vi "Day 8 - Haunted Wasteland.vi"() -> ()   [LabVIEW 2020, in "AoC 2023.lvlib"]
uses:
  AoC 2023.lvlib
  0a6171a5-c240-4508-9ae7-3547d43446d7.vi
  <vilib>/gmath/NI_AAL_MathFunc.lvlib
panel:
  out "Puzzle Part-2 Answer":string
  out "Puzzle Answer":string
  in  "Puzzle Input":string="RL\n\nAAA = (BBB, CCC)\nBBB = (DDD, EEE)\nCCC = (ZZZ, GGG)\nDDD = (DDD, DDD)\nEEE = (EEE, EEE)\nGGG = (GGG, GGG)\nZZZ = (ZZZ, ZZZ)"
  # "Enter the Puzzle Input and run the VI"
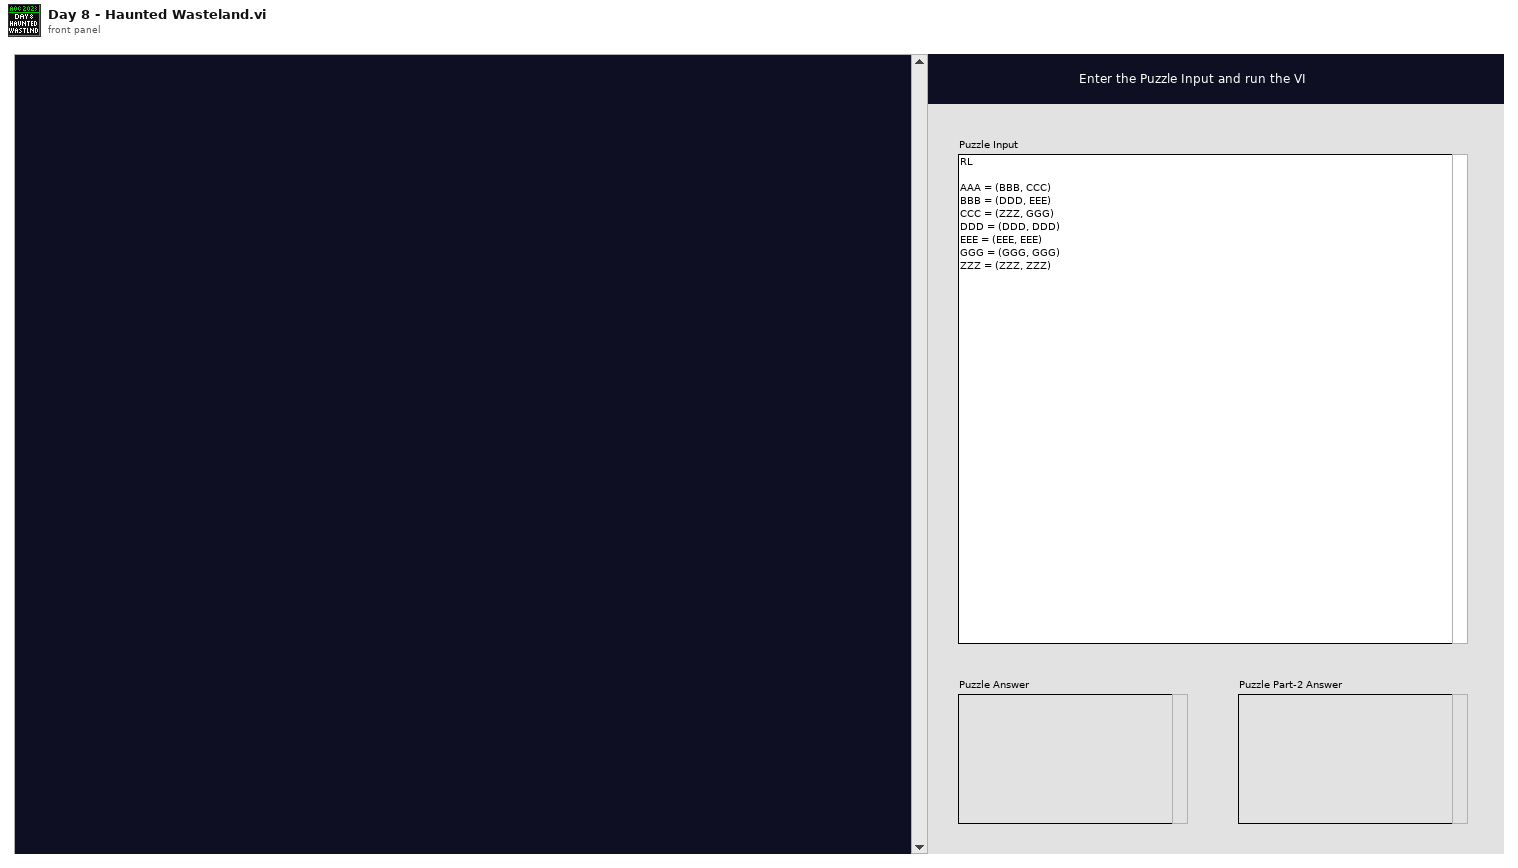
[diagram p1: front panel]
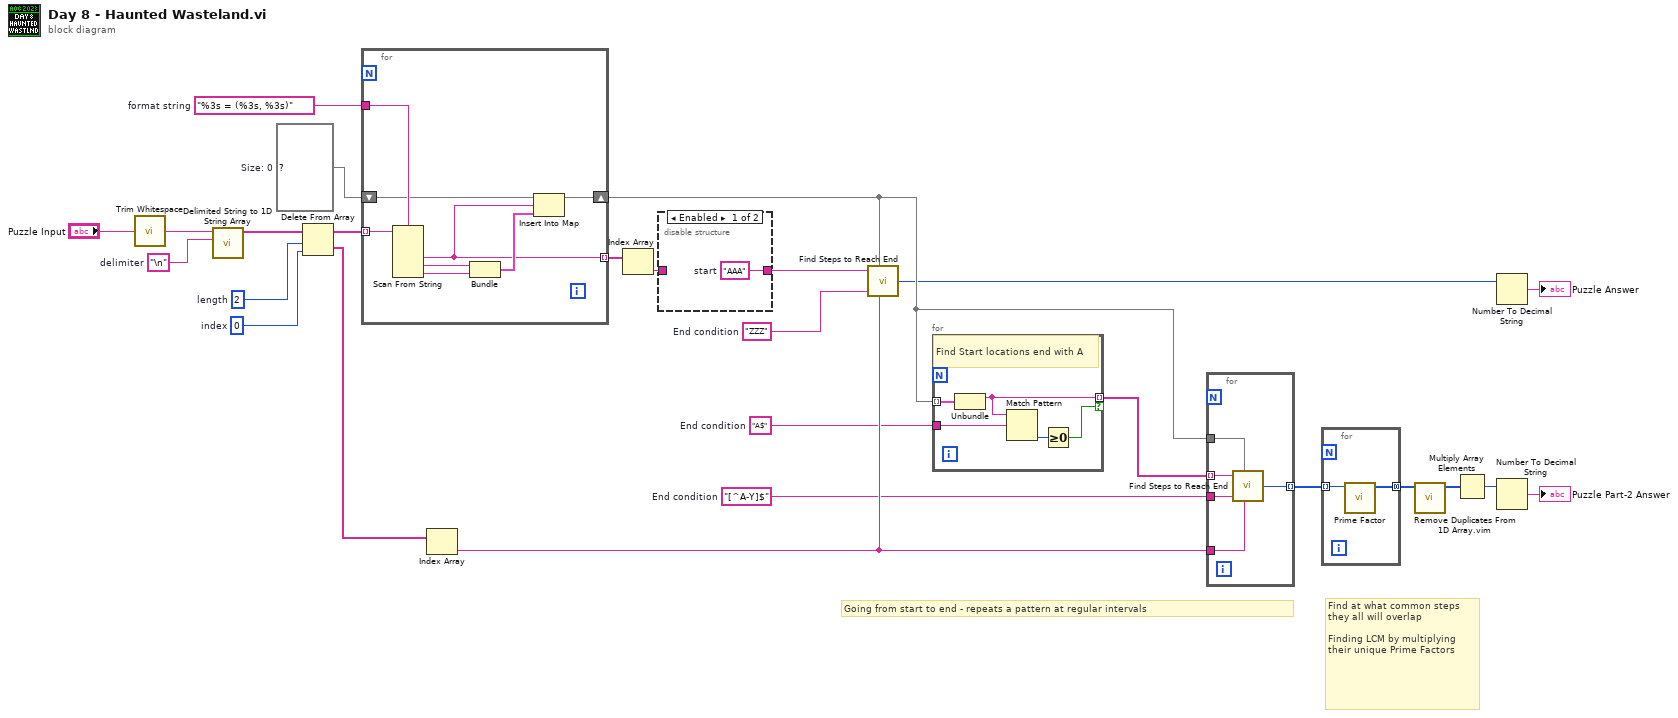
[diagram p0: block diagram]
diagram:
  w8 = "A$"  # End condition
  w9 = "[^A-Y]$"  # End condition
  w11 = "ZZZ"  # End condition
  w16 = map{string, cluster{string, string}} {}  # Size: 0
  w17 = 2  # length
  w18 = 0  # index
  w22 = "%3s = (%3s, %3s)"  # format string
  w23 = "\n"  # delimiter
  # "Find at what common steps they all will overlap\n\nFinding LCM by multiplying their unique Prime Factors"
  # "Going from start to end - repeats a pattern at regular intervals"
  n1 = call <vilib>:"Trim Whitespace.vi"("string"="Puzzle Input") -> ("trimmed string"=w21:string)  [unwired: 1 in]
  n2 = call <vilib>:"Delimited String to 1D String Array.vi"("delimiter"=w23, "delimited string"=w21) -> ("string array"=w20:string[])  [unwired: 9 in]
  n3 = Delete From Array(array=w20, length=w17, index=w18) -> (deleted portion=w12:string[], array with subset deleted=w19:string[])
  n4 = for {
    tunnel: w19 -> [w34] mode=indexing
    tunnel: w22 -> [w33]
    shift-right: [w29] -> w6
    shift-left: w16 -> [w28]
    tunnel: [w27] -> w15 mode=indexing
    n5 = Scan From String(format string=w33, input string=w34) -> (output 1=w27:string, output 2=w32:string, output 3=w31:string)  [unwired: 5 in, 3 out]
    n6 = Bundle(w32, w31) -> (w30:cluster{string, string})  [unwired: 1 in]
    n7 = Insert Into Map(map in=w28, key=w27, value=w30) -> (map out=w29:map{string, cluster{string, string}})  [unwired: 2 out]
  }
  n8 = Index Array(array=w12) -> (element=w10:string)  [unwired: 1 in]
  n9 = Index Array(array=w15) -> (element=w14:string)  [unwired: 1 in]
  n10 = disable-structure shown="Enabled" {
    disable-tunnel: [w35 w36] -> w13
    disable-tunnel: w14 -> [_ w36]
    frame Enabled {
      w35 = "AAA"  # start
    }
    frame Disabled {
      # "bug"
    }
  }
  n11 = call "Find Steps to Reach End.vi"("Start position"=w13, "Map"=w6, "End condition"=w11, "Instructions"=w10) -> ("Steps to reach last end"=w5:u64)  [unwired: 4 in, 1 out]
  n12 = for {
    tunnel: w6 -> [w41] mode=indexing
    tunnel: w8 -> [w39]
    tunnel: [w38] -> w7 mode=indexing if=w37
    # "Find Start locations end with A"
    n13 = Unbundle(w41) -> (w38:string)  [unwired: 1 out]
    n14 = Match Pattern(string=w38, regular expression=w39) -> (offset past match=w40:i32)  [unwired: 1 in, 3 out]
    n15 = Greater Or Equal To 0?(x=w40) -> (x >= 0?=w37:bool)
  }
  n16 = for {
    tunnel: w10 -> [w46]
    tunnel: [w45] -> w4 mode=indexing
    tunnel: w6 -> [w44]
    tunnel: w9 -> [w43]
    tunnel: w7 -> [w42] mode=indexing
    n17 = call "Find Steps to Reach End.vi"("Start position"=w42, "Map"=w44, "End condition"=w43, "Instructions"=w46) -> ("Steps to reach last end"=w45:u64)  [unwired: 4 in, 1 out]
  }
  n18 = for {
    tunnel: w4 -> [w48] mode=indexing
    tunnel: [w47] -> w3 mode=concatenating
    n19 = call <vilib>:"Prime Factor.vi"("n"=w48) -> ("Prime Factors"=w47:i64[])  [unwired: 9 in]
  }
  n20 = call "Remove Duplicates From 1D Array.vim"("array"=w3) -> ("array with duplicates removed"=w2:i64[])  [unwired: 10 in]
  n21 = Multiply Array Elements(1:w2) -> (0:w1:i64)
  n22 = Number To Decimal String(number=w5) -> (decimal integer string=→"Puzzle Answer":string)  [unwired: 1 in]
  n23 = Number To Decimal String(number=w1) -> (decimal integer string=→"Puzzle Part-2 Answer":string)  [unwired: 1 in]
